vi "Store_Results.vi"(10 "Positions in":T1(array[cluster]) {"Error Code" format="%b"; "ID" format="%x"}, 11 "Joint Info":T2 {"Error Code" format="%b"; "ID" format="%x"}) -> (3 "Stored positions":T1(array[cluster]) {"Error Code" format="%b"; "ID" format="%x"})   [LabVIEW 2015]
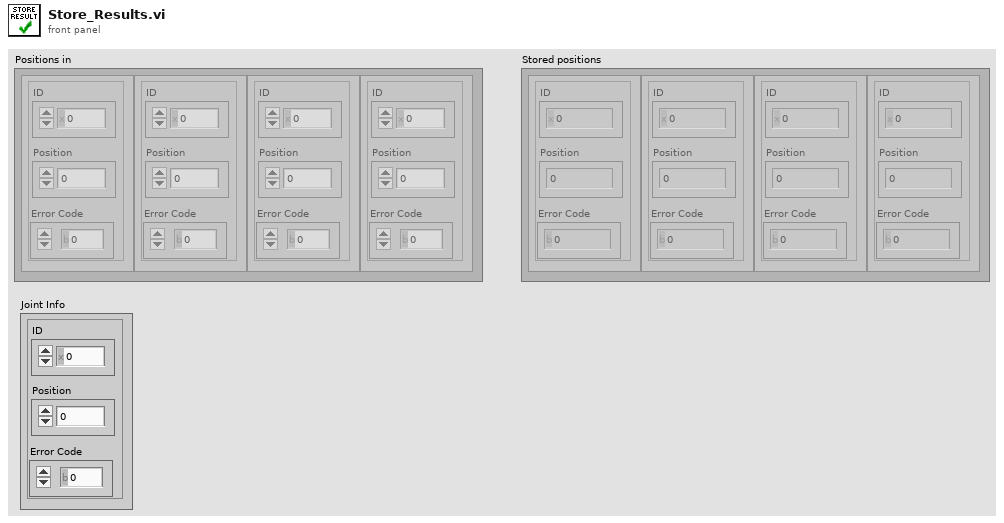
[diagram p1: front panel]
types:
  T1 = cluster{"ID":u8, "Position":u16, "Error Code":u8}[]
  T2 = cluster{"ID":u8, "Position":u16, "Error Code":u8}
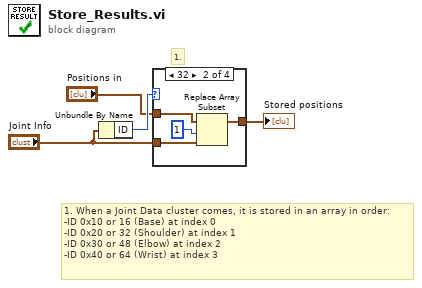
[diagram p0: block diagram]
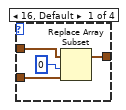
[diagram p2: hidden frame]
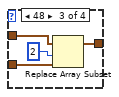
[diagram p3: hidden frame]
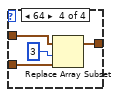
[diagram p4: hidden frame]
diagram:
  # "1."
  # "1. When a Joint Data cluster comes, it is stored in an array in order:\n-ID 0x10 or 16 (Base) at index 0\n-ID 0x20 or 32 (Shoulder) at index 1\n-ID 0x30 or 48 (Elbow) at index 2\n-ID 0x40 or 64 (Wrist) at index 3"
  n1 = Unbundle By Name("Joint Info") -> ("ID"=w4:u8)
  n2 = case shown="32" w4 {
    tunnel: "Joint Info" -> [w6 w10 w14 w20]
    tunnel: "Positions in" -> [w7 w11 w15 w19]
    tunnel: [w5 w9 w13 w17] -> w1
    frame 16, Default {
      n3 = Replace Array Subset(array=w7, new element=w6, index=0) -> (w5:T1)
    }
    frame 32 {
      n4 = Replace Array Subset(array=w11, new element=w10, index=1) -> (w9:T1)
    }
    frame 48 {
      n5 = Replace Array Subset(array=w15, new element=w14, index=2) -> (w13:T1)
    }
    frame 64 {
      n6 = Replace Array Subset(array=w19, new element=w20, index=3) -> (w17:T1)
    }
  }
  "Stored positions" <- w1
